vi "Select PCB quality.vi"(8 "error in (no error)":errorcluster, 9 "Bypass查詢":bool, 10 "barcode":string="搜尋條件", 11 "DBlink":string="Driver={ODBC Driver 17 for SQL Server};Server=localhost\\SQLEXPRESS;Database=YDXB01;UID=labview;PWD=123456789") -> (0 "error out":errorcluster={"status"=TRUE, "code"=-2147217900, "source"="NI_Database_API.lvlib:Conn Execute.vi->NI_Database_API.lvlib:DB Tools Select Data.vi->Select WebCam BBOX.vi<ERR>ADO Error: 0x80040E14\r\nException occured in Microsoft OLE DB Provider for ODBC Drivers: [Microsoft][ODBC Driver 17 for SQL Server][SQL Server]接近 ',' 之處的語法不正確。 in NI_Database_API.lvlib:Conn Execute.vi->NI_Database_API.lvlib:DB Tools Select Data.vi->Select WebCam BBOX.vi"}, 2 "result":string, 3 "size(s)":i32)   [LabVIEW 2019]
uses:
  <vilib>/addons/database/Connection.llb/DB Tools Open Connec (String).vi
  <vilib>/addons/database/_DB Variant To Data/Database Variant To Data.xnode
  <vilib>/addons/database/NI_Database_API.lvlib
panel:
  in  "table":string="指定資料表"
  out "data":cluster{string}[](array[cluster])
  out "sql command":string="where barcode='400010505'  and box = 'B'  and depth = 1000"
  in  "columns":string[](array[string])=["結果欄位"]
  # "True為OK"
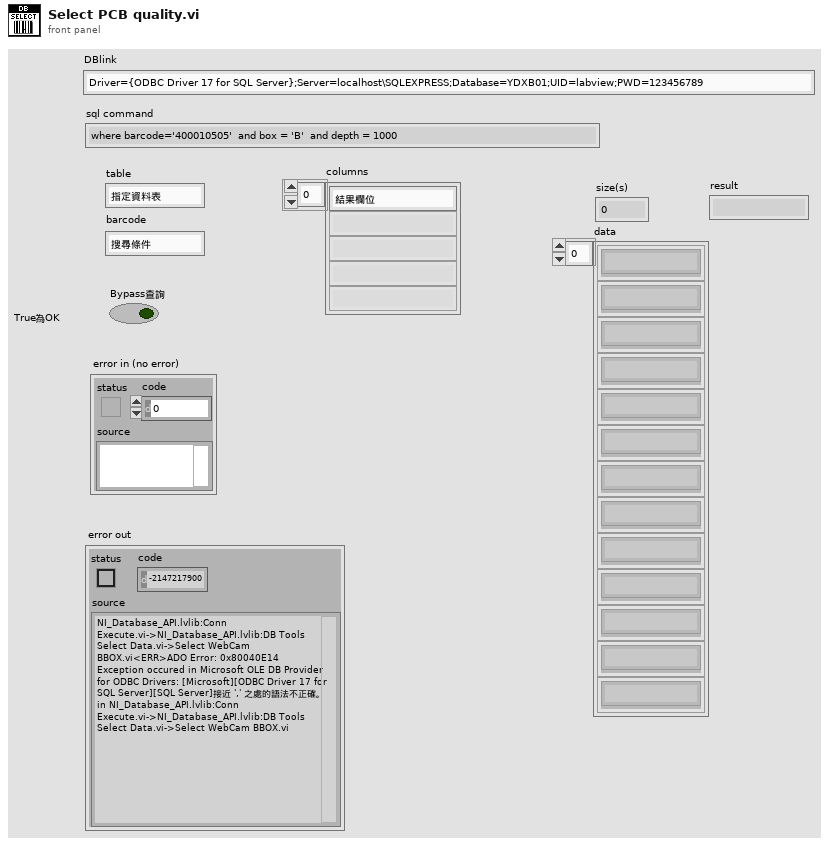
[diagram p1: front panel]
types:
  T1 = typedef "NI_Database_API.lvlib/Conn ObjectReference.ctl" = refnum<k1>
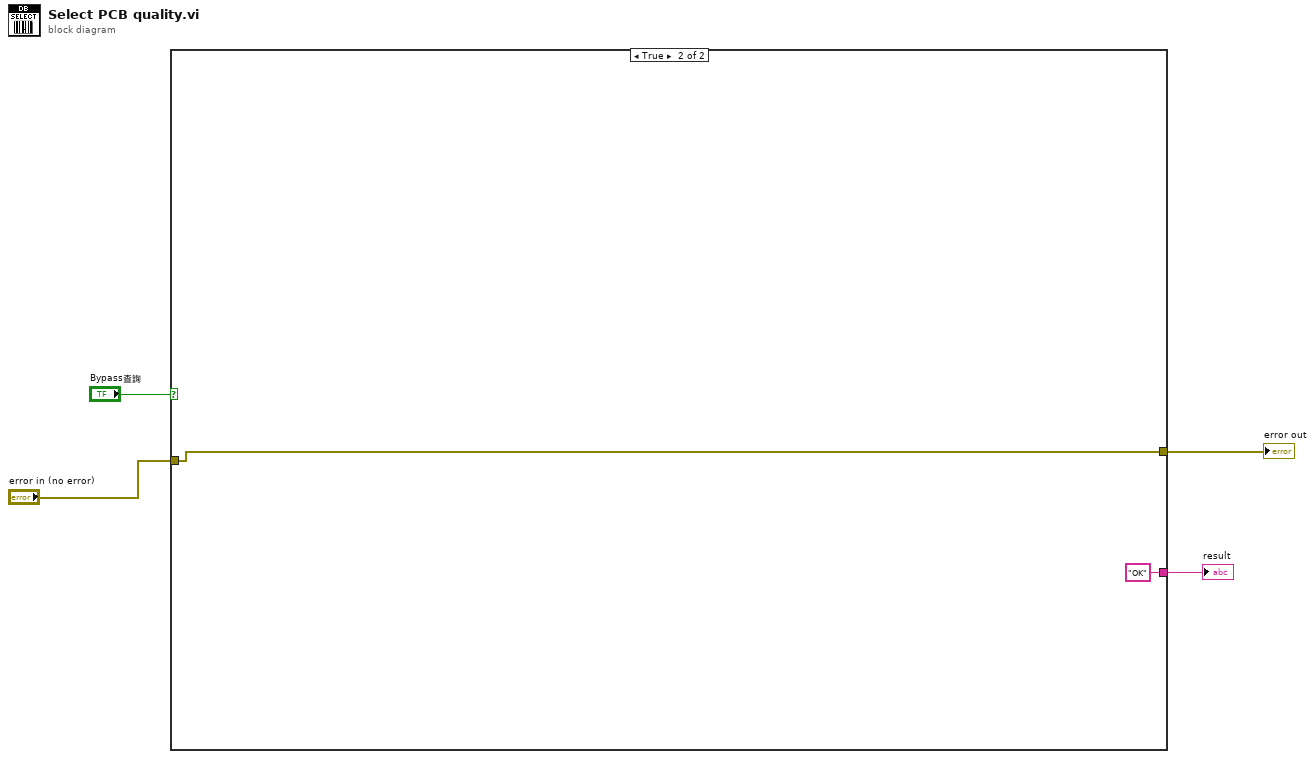
[diagram p0: block diagram]
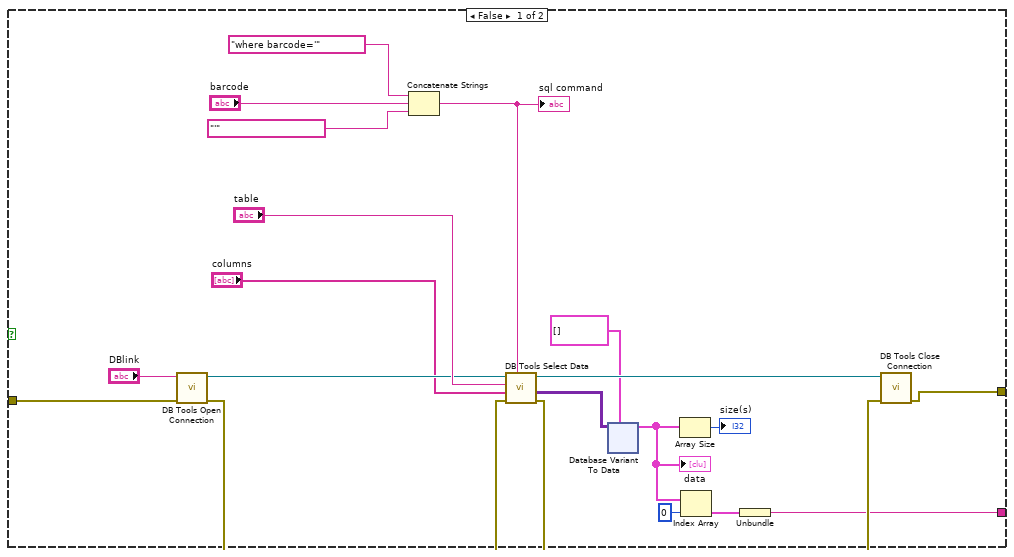
[diagram p2: hidden frame]
diagram:
  n1 = case shown="True" "Bypass查詢" {
    tunnel: [w7 "OK"] -> w4
    tunnel: "error in (no error)" -> [w6 w66]
    tunnel: [w5 w66] -> w1
    frame False {
      n2 = call-poly <vilib>:"DB Tools Open Connection.vi"("error in (no error)"=w6, "connection information"="DBlink") -> ("error out"=w21:errorcluster, "connection reference"=w22:T1)  [unwired: 6 in]
      n3 = Concatenate Strings("where barcode='" ("format string"), "barcode", "'" ("format string")) -> (w15:string)
      "sql command" <- w15
      n4 = call <vilib>:"DB Tools Select Data.vi"("condition"=w15, "error in (no error)"=w21, "columns"="columns", "table"="table", "connection reference"=w22) -> ("error out"=w19:errorcluster, "data"=w12:variant[][], "connection reference out"=w20:T1)  [unwired: 1 in]
      n5 = xnode "Database Variant To Data"("database variant"=w12, "type"=cluster{"result":string}[] [] ("Region number")) -> ("data"=w10:cluster{string}[])  [unwired: 1 in, 1 out]
      "data" <- w10
      n6 = Array Size(array=w10) -> (size(s)=→"size(s)":i32)
      n7 = Index Array(array=w10, index=0) -> (element=w8:cluster{string})
      n8 = Unbundle(w8) -> (w7:string)
      n9 = call <vilib>:"DB Tools Close Connection.vi"("error in (no error)"=w19, "connection reference"=w20) -> ("error out"=w5:errorcluster)  [unwired: 5 in]
    }
    frame True {
    }
  }
  "result" <- w4
  "error out" <- w1
